vi "Get SMO Public API.vi"(8 "error in (no error)":errorcluster, 11 "Instrument.Example In":refnum<class "Instrument.Oxford1820.lvclass">) -> (0 "error out":errorcluster, 2 "Commands":string[](array[string]), 3 "Instrument.Example out":refnum<class "Instrument.Oxford1820.lvclass">)   [LabVIEW 2019, in "Instrument.Oxford1820.lvclass"]
uses:
  Instrument.Oxford1820.lvclass
  C:/Program Files (x86)/National Instruments/LabVIEW 2019/user.lib/LevyLab/Instrument Framework/Instrument/Instrument.lvclass
  Typedefs/Instrument.Oxford1820.publicCommands-enum.ctl
  <userlib>/LevyLab/Instrument Framework/Instrument Types/Cryostat/Instrument.Cryostat.lvclass
  <userlib>/LevyLab/Instrument Framework/Instrument/Instrument.lvclass
panel:
  in  "Commands":T1
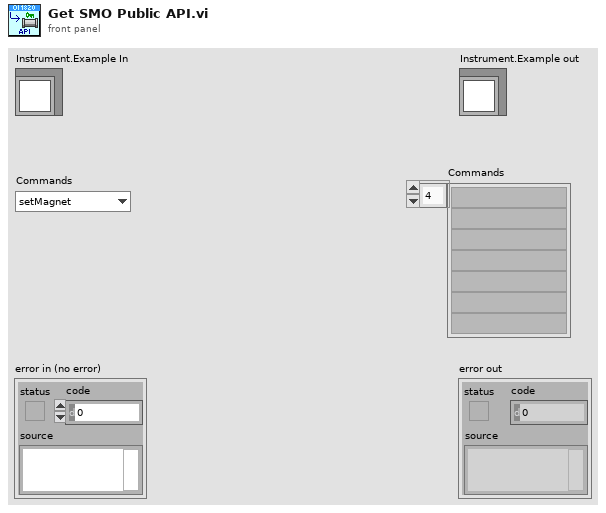
[diagram p1: front panel]
types:
  T1 = typedef "Instrument.Oxford1820.lvclass/Instrument.Oxford1820.publicCommands-enum.ctl" = enum16{"setMagnet", "getMagnet", "getMagnetTarget", "getHeLevel", "getN2level"}
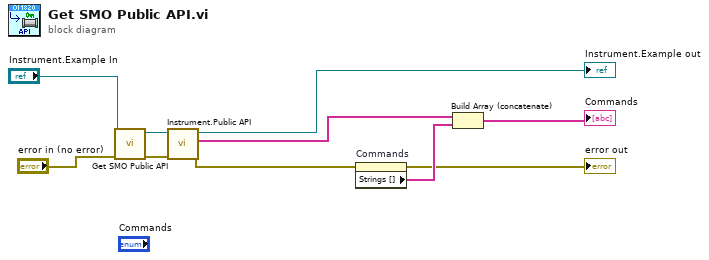
[diagram p0: block diagram]
diagram:
  n1 = call-parent "Get SMO Public API.vi"("error in (no error)"="error in (no error)", "Instrument.Cryostat in"="Instrument.Example In") -> ("error out"=w4:errorcluster, "Instrument.Cryostat out"=w2:refnum<class "Instrument.Oxford1820.lvclass">)  [unwired: 7 in, 1 out]
  n2 = call <userlib>:"Instrument.Public API.vi"("error in (no error)"=w4, "Instrument in"=w2) -> ("error out"=w3:errorcluster, "commands (this level)"=w5:string[], "Instrument out"=→"Instrument.Example out":refnum<class "Instrument.Oxford1820.lvclass">)  [unwired: 7 in]
  n3 = property on="Commands" class="Enum (strict)"(error in=w3) -> (error out=→"error out":errorcluster, "Strings []"=w7:string[])  [unwired: 1 in, 1 out]
  n4 = Build Array (concatenate)(w5, w7) -> (→"Commands":string[])
